vi "HEWH Cut Power.vi"(9 "Cut Power At Time (Sec)":T1 format="%<%H:%M:%S>t", 10 "Current Draw Time (Sec)":T1 format="%<%H:%M:%S>t", 11 "User Controls in":T2={"Main Power Control"=FALSE, "Flow Totalizer Control"=FALSE, "Intellifaucet \nTemperature"=0.0, "Percent Flow"=0.0, "Safe Mode"=FALSE, "GEA2?"=FALSE, "Use Agilent?"=FALSE, "Valve Set A"=enum."Heating", "Valve Set B"=enum."Heating", "Valve Set C"=enum."Heating", "Valve Set D"=enum."Heating", "Valve Ctrl"={"Outlet Valve D"="OFF", "Drain Valve D"="OFF", "Inlet Valve D"="ON", "Outlet Valve C"="OFF", "Drain Valve C"="OFF", "Inlet Valve C"="ON", "Outlet Valve B"="OFF", "Drain Valve B"="OFF", "Inlet Valve B"="ON", "Outlet Valve A"="OFF", "Drain Valve A"="OFF", "Inlet Valve A"="ON"}, "Proportional Valve"=1.0, "Reset Auto Step"=FALSE} {"Proportional Valve" scale=0.0..100.0; "Percent Flow" scale=0.0..100.0; "Intellifaucet \nTemperature" scale=40.0..120.0}) -> (2 "States Output":string, 3 "User Controls out":T2={"Main Power Control"=FALSE, "Flow Totalizer Control"=FALSE, "Intellifaucet \nTemperature"=0.0, "Percent Flow"=0.0, "Safe Mode"=FALSE, "GEA2?"=FALSE, "Use Agilent?"=FALSE, "Valve Set A"=enum."Heating", "Valve Set B"=enum."Heating", "Valve Set C"=enum."Heating", "Valve Set D"=enum."Heating", "Valve Ctrl"={"Outlet Valve D"="OFF", "Drain Valve D"="OFF", "Inlet Valve D"="ON", "Outlet Valve C"="OFF", "Drain Valve C"="OFF", "Inlet Valve C"="ON", "Outlet Valve B"="OFF", "Drain Valve B"="OFF", "Inlet Valve B"="ON", "Outlet Valve A"="OFF", "Drain Valve A"="OFF", "Inlet Valve A"="ON"}, "Proportional Valve"=1.0, "Reset Auto Step"=FALSE} {"Proportional Valve" scale=0.0..100.0; "Percent Flow" scale=0.0..100.0; "Intellifaucet \nTemperature" scale=40.0..120.0})   [LabVIEW 2019]
uses:
  Type Definitions/HEWH User Controls.ctl
  Type Definitions/HEWH Normally Open Valve Control.ctl
  Type Definitions/HEWH Normally Closed Valve Control.ctl
  Utility/Custom Pallet Controls/Custom Pallet Timer.ctl
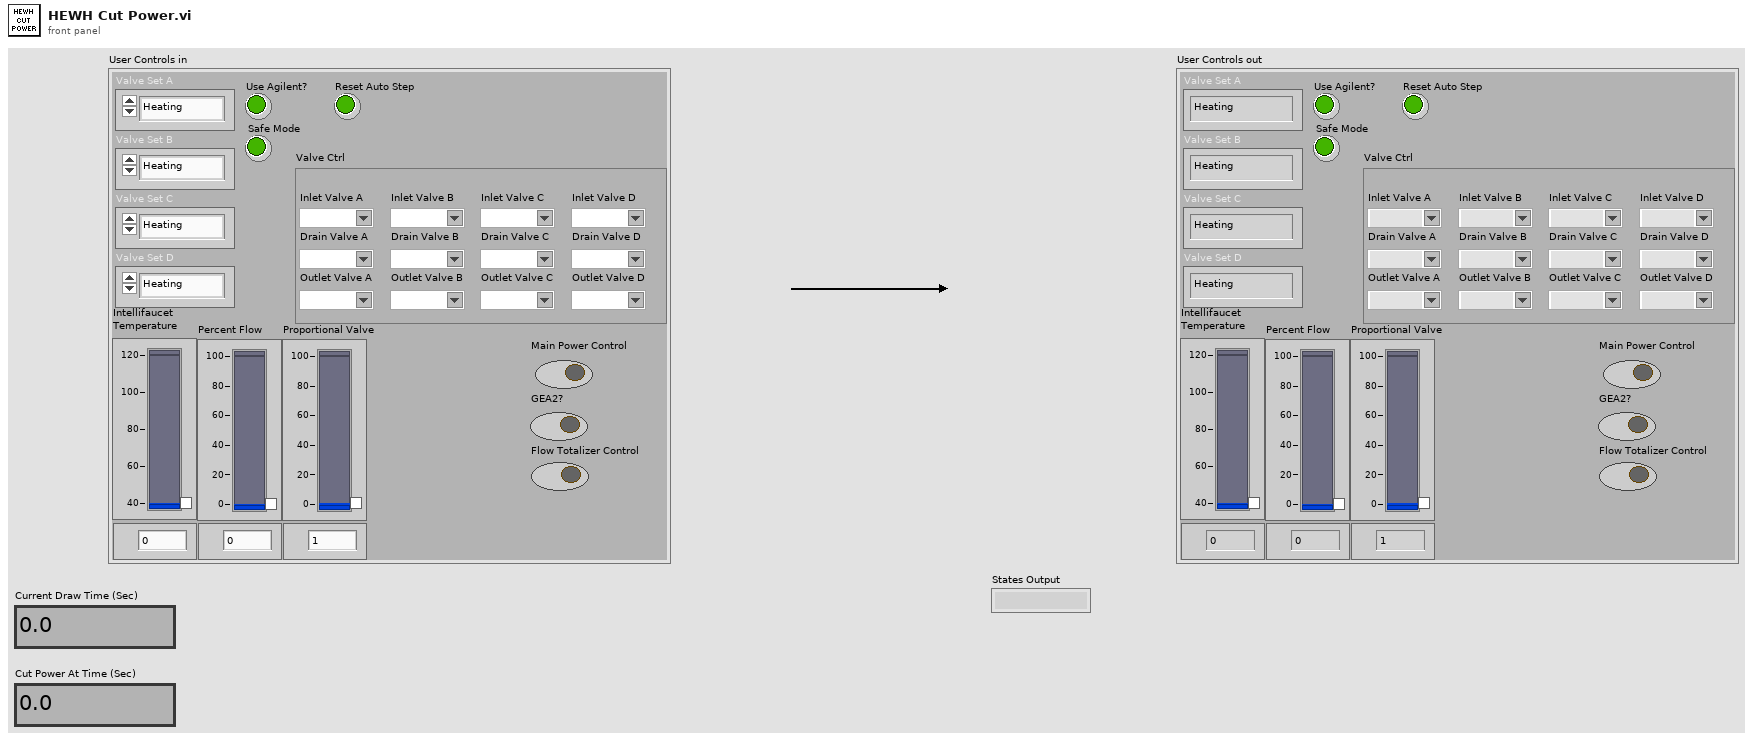
[diagram p1: front panel]
types:
  T1 = typedef "Custom Pallet Timer.ctl" = dbl
  T2 = typedef "HEWH User Controls.ctl" = cluster{"Main Power Control":bool, "Flow Totalizer Control":bool, "Intellifaucet \nTemperature":dbl, "Percent Flow":dbl, "Safe Mode":bool, "GEA2?":bool, "Use Agilent?":bool, "Valve Set A":enum16{"Heating", "Purge", "Resting", "Draw"}, "Valve Set B":enum16{"Heating", "Purge", "Resting", "Draw"}, "Valve Set C":enum16{"Heating", "Purge", "Resting", "Draw"}, "Valve Set D":enum16{"Heating", "Purge", "Resting", "Draw"}, "Valve Ctrl":cluster{"Outlet Valve D":T3, "Drain Valve D":T4, "Inlet Valve D":T3, "Outlet Valve C":T3, "Drain Valve C":T4, "Inlet Valve C":T3, "Outlet Valve B":T3, "Drain Valve B":T4, "Inlet Valve B":T3, "Outlet Valve A":T3, "Drain Valve A":T4, "Inlet Valve A":T3}, "Proportional Valve":dbl, "Reset Auto Step":bool}
  T3 = typedef "HEWH Normally Open Valve Control.ctl" = string
  T4 = typedef "HEWH Normally Closed Valve Control.ctl" = string
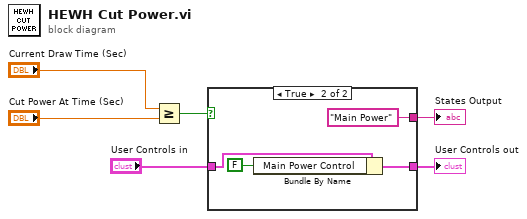
[diagram p0: block diagram]
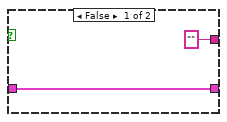
[diagram p2: hidden frame]
diagram:
  n1 = Greater Or Equal?(x="Current Draw Time (Sec)", y="Cut Power At Time (Sec)") -> (x >= y?=w3:bool)
  n2 = case shown="True" w3 {
    tunnel: ["" ("State(s) in Front (\"\")") "Main Power" ("State(s) in Front (\"\")")] -> w4
    tunnel: "User Controls in" -> [w7 w11]
    tunnel: [w7 w10] -> w6
    frame False {
    }
    frame True {
      n3 = Bundle By Name(cluster=w11, "Main Power Control"=FALSE ("User Controls.Main Power Control")) -> (w10:T2)
    }
  }
  "User Controls out" <- w6
  "States Output" <- w4
